vi "gyro-sweeper-server-V3.vi"(11 "talk to back IN":T4) -> ()   [LabVIEW 2018]
uses:
  cursor winow.ctl
  cursor window action.ctl
  KM_file -- read-write control.ctl
  filename-action.ctl
  file -- read-write control.ctl
  publisher action.ctl
  show-win- control.ctl
  data source action.ctl
  pll user action.ctl
  pll sweeper talkto message type.ctl
  pll sweeper talkback message type.ctl
  pll fitter talkto message type.ctl
  pll fitter talkback message type.ctl
  pll sweeper server talkto message type.ctl
  pll sweeper server talkback message type.ctl
  pll talkback message type.ctl
  filename-pattern.ctl
  talkto talkback pair.ctl
panel:
  out "Stop":bool
  in  "view/hide fitter async":bool
  in  "view/hide sweep async":bool
  in  "sweeper panel":T1(tab)
  in  "sweep ON":bool
  in  "win":T2={"cen (Hz)"=45005.0594236074, "win (Hz)"=127.23590686512762, "left (Hz)"=44941.44147017484, "right (Hz)"=45068.67737703997}
  out "Plot: circle sweep window":cluster{"Freq out (Hz)":dbl[], dbl[]}[](graph)
  in  "start/stop sweep: r":bool
  in  "subtract bgnd!":bool
  in  "fit!":bool=TRUE
  in  "cursor window":T3={"left"=2378.60310421286, "right "=2421.6740576496672, "center"=2421.6740576496672, "window"=2421.6740576496672, "cursors"=[], "relative"=0, "absolute"=0, "fixed vertical offset"=2421.6740576496672, "vertical offset"=2421.6740576496672, "skew"=2421.6740576496672, "default window frac"=2421.6740576496672, "kind"=enum."skewed", "skew.left"=2421.6740576496672, "skew.right"=2421.6740576496672, "Plot ref"=refnum, "wing order"=enum."back"}
  out "async sweeper reference out":refnum<vi>
  out "async fitter":refnum<vi>
  in  "save data":enum32{"save/read"}(tab)
  in  "freqsweep name template":T5={"prefix"="RuCl3-rod", "group"="f"}
  in  "Save folder":path=path "/Users/Shared/Data"
  in  "freq sweep file name":string="f020_RuCl3-rod_042518.dat"
  in  "read from disk :l":bool
  in  "read file":path=path "/Users/arkady/Desktop/local_data/TaAs-quirk-Jan2018-losalamos/9w/f006_rucl3_012518.dat"
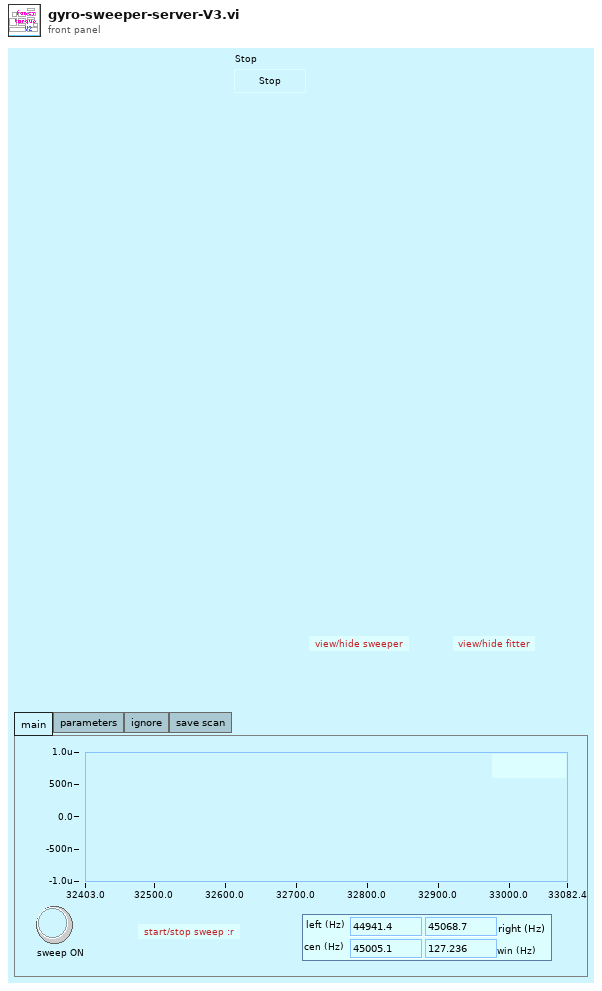
[diagram p1: front panel]
types:
  T1 = enum32{"main", "parameters", "ignore", "save scan"}
  T2 = typedef "show-win- control.ctl" = cluster{"cen (Hz)":dbl, "win (Hz)":dbl, "left (Hz)":dbl, "right (Hz)":dbl}
  T3 = typedef "cursor winow.ctl" = cluster{"left":dbl, "right ":dbl, "center":dbl, "window":dbl, "cursors":i32[], "relative":i32, "absolute":i32, "fixed vertical offset":dbl, "vertical offset":dbl, "skew":dbl, "default window frac":dbl, "kind":enum16{"symmetric", "skewed", "fancy"}, "skew.left":dbl, "skew.right":dbl, "Plot ref":refnum<vi>, "wing order":enum16{"forw", "back"}}
  T4 = typedef "talkto talkback pair.ctl" = cluster{"talkto event":refnum<user-event>, "talkback event":refnum<user-event>}
  T5 = typedef "filename-pattern.ctl" = cluster{"prefix":string, "group":string}
  T6 = cluster{"talkto event":refnum<user-event>, "talkback event":refnum<user-event>}
  T7 = typedef "pll fitter talkback message type.ctl" = cluster{"message":enum16{"new "}}
  T8 = typedef "pll fitter talkto message type.ctl" = cluster{"message":enum16{"stop", "start", "get new"}}
  T9 = typedef "data source action.ctl" = enum16{"set", "get", "init", "set-and-get", "init source"}
  T10 = typedef "pll sweeper talkback message type.ctl" = cluster{"message":enum16{"new"}}
  T11 = typedef "pll sweeper talkto message type.ctl" = cluster{"message":enum16{"stop", "start", "update pars"}}
  T12 = typedef "pll user action.ctl" = enum16{"fit"}
  T13 = typedef "publisher action.ctl" = enum16{"set", "get", "init", "check"}
  T14 = typedef "cursor window action.ctl" = enum16{"balance", "h. offset change", "cursor moves", "change center", "change window", "init", "check", "reset", "set y to middle", "idle", "-write all Y", "-write left.X", "-write center.X", "-write right.X", "-write all X", "-change center", "-change window", "-change skew", "-read cursor 2", "-read cursor 1", "-read cursor 0", "-read all cursors", "-reset", "-read plot scale", "-set y to middle", "-Q: center.Y is visible", "-Q: window is visible", "-parse center.Y", "-right left from center", "-left move", "-right move", "-set center.Y", "-empty", "-set cursors to default", "-check", "-write center.Y", "-copy cursor 1", "-copy cursor 0", "-copy cursor 2", "move right", "move left", "shrink", "broaden", "skew up", "skew down", "-write plot scale", "zoom X", "change cen&win", "zoom to all data", "color--red", "color--green", "color--yellow", "read", "zoom out", "zoom in", "slide right", "slide left", "set range aspect ratio to 1"}
  T15 = typedef "PLL data source.ctl" = enum16{"meta", "MFLI", "SRS865A"}
  T16 = typedef "file -- read-write control.ctl" = enum16{"read", "write all", "append one line"}
  T17 = typedef "filename-action.ctl" = enum16{"rewrite", "parse", "force pattern", "uniquenum"}
  T18 = typedef "KM_file -- read-write control.ctl" = enum16{"read", "write all", "append one line"}
  T19 = enum32{"Invalid", "Standard", "Closed", "Hidden", "Minimized", "Maximized"}
  T20 = typedef "eventvkey.ctl" = enum16{"ASCII", "Enter", "Return", "Shift", "Ctrl", "Alt", "Cmd", "Opt", "Caps", "NumLock", "Clear", "Break", "Up", "Down", "Left", "Right", "Insert", "Delete", "Home", "End", "PageUp", "PageDown", "Escape", "Help", "Pause", "ScrollLock", "F1", "F2", "F3", "F4", "F5", "F6", "F7", "F8", "F9", "F10", "F11", "F12", "F13", "F14", "F15", "F16", "F17", "F18", "F19", "F20", "F21", "F22", "F23", "F24", "Play", "VolumeUp", "VolumeDown", "Mute", "Two Byte Char"}
  T21 = typedef "pll talkback message type.ctl" = cluster{"message":enum16{"new", ""}}
  T22 = enum16{"exit", "parameter change", "start", "stop", "reset frequency", "reset lorentzian"}
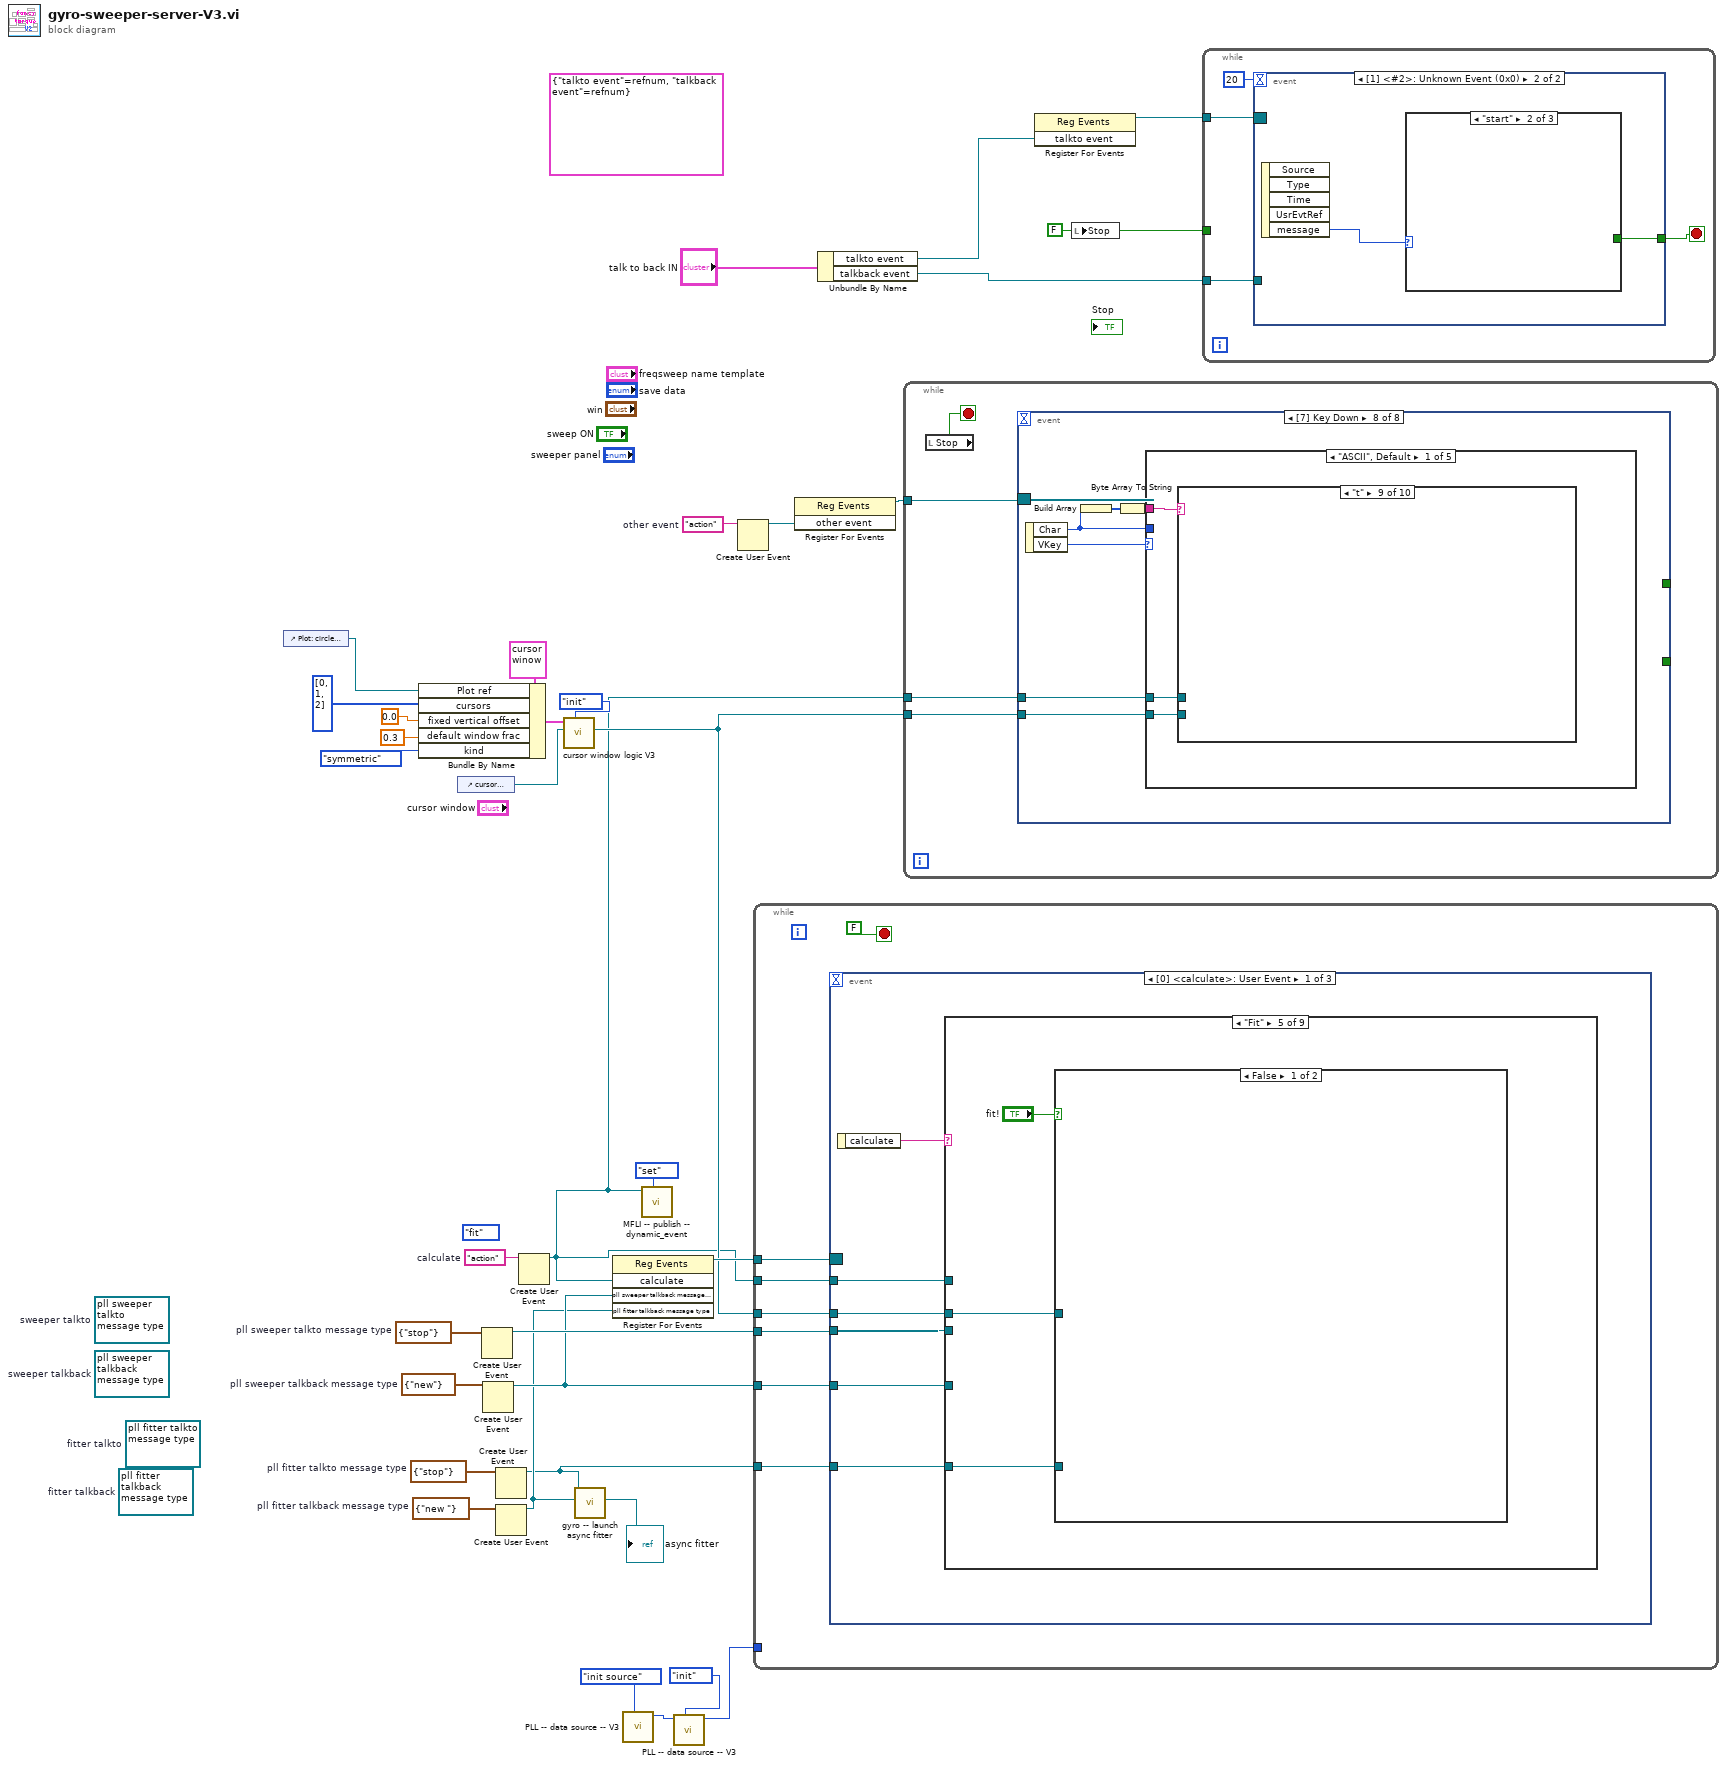
[diagram p0: block diagram]
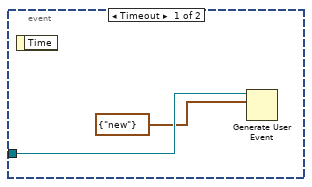
[diagram p2: hidden frame]
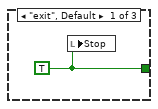
[diagram p3: hidden frame]
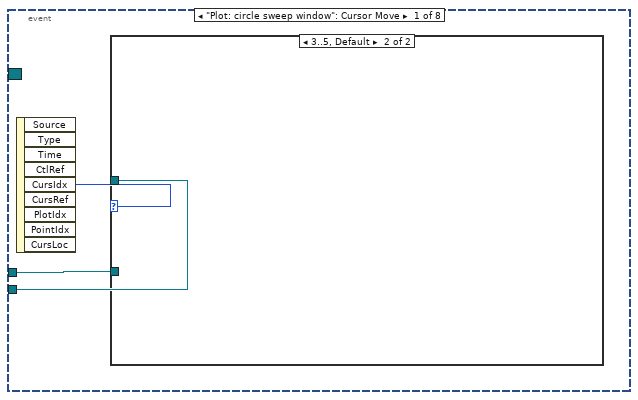
[diagram p5: hidden frame]
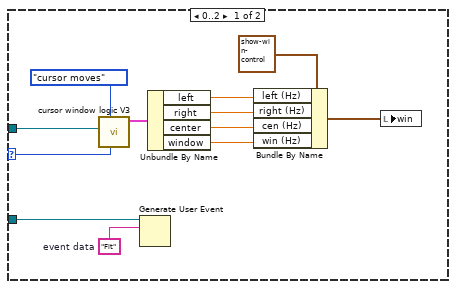
[diagram p6: hidden frame]
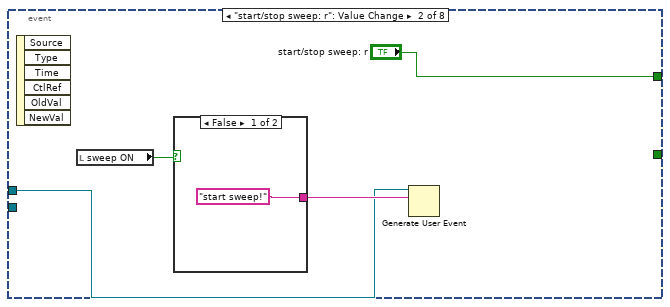
[diagram p7: hidden frame]
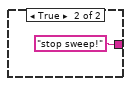
[diagram p8: hidden frame]
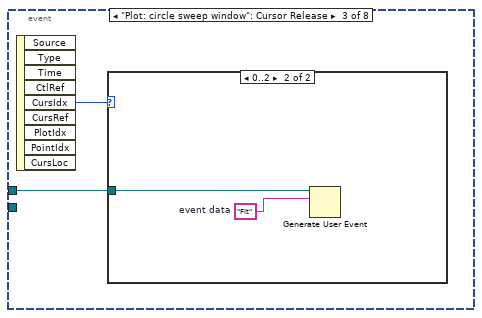
[diagram p9: hidden frame]
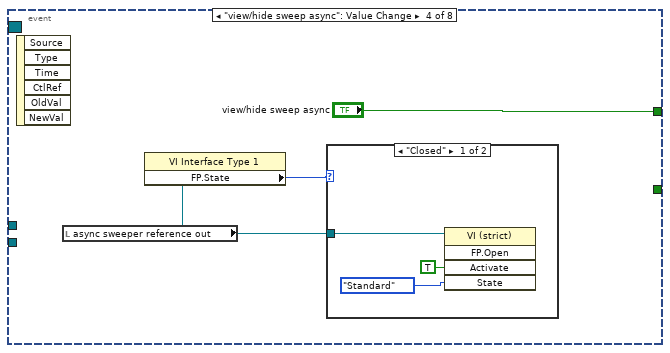
[diagram p11: hidden frame]
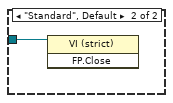
[diagram p12: hidden frame]
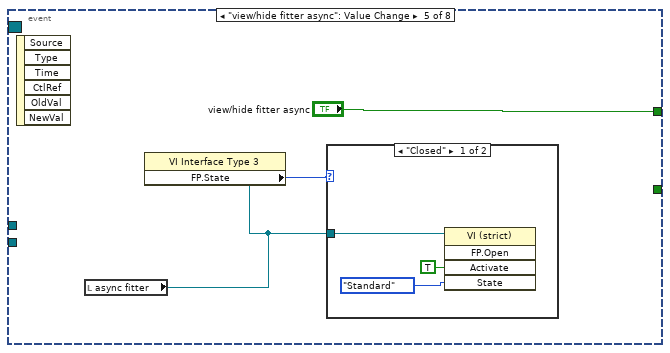
[diagram p13: hidden frame]
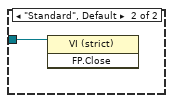
[diagram p14: hidden frame]
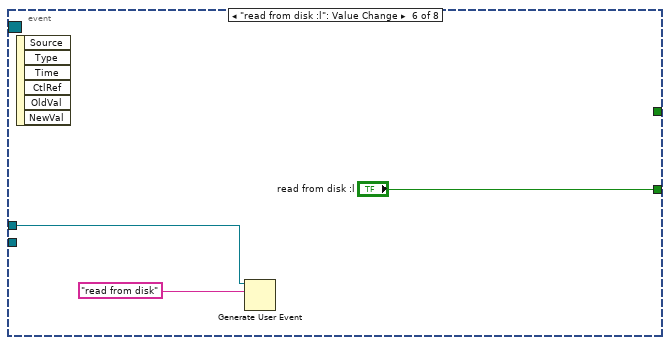
[diagram p15: hidden frame]
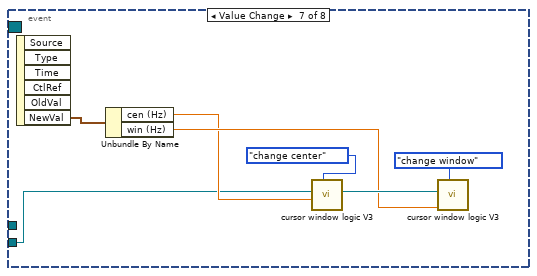
[diagram p16: hidden frame]
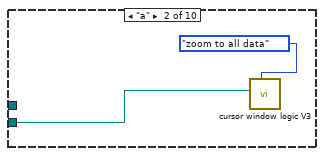
[diagram p18: hidden frame]
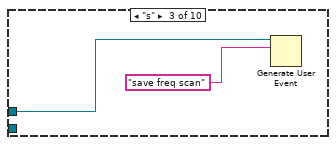
[diagram p19: hidden frame]
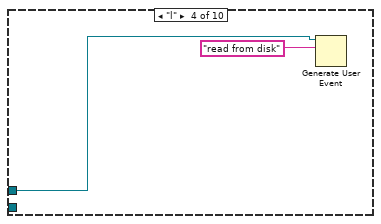
[diagram p20: hidden frame]
diagram:
  w4 = FALSE ("Stop")
  (unwired) T6 {"talkto event"=refnum, "talkback event"=refnum}
  (unwired) refnum<user-event> refnum  # fitter talkback
  (unwired) refnum<user-event> refnum  # fitter talkto
  w11 = T7 {"message"=enum."new "}  # pll fitter talkback message type
  w10 = T8 {"message"=enum."stop"}  # pll fitter talkto message type
  (unwired) refnum<user-event> refnum  # sweeper talkback
  (unwired) refnum<user-event> refnum  # sweeper talkto
  w19 = T10 {"message"=enum."new"}  # pll sweeper talkback message type
  w20 = T11 {"message"=enum."stop"}  # pll sweeper talkto message type
  (unwired) pll_user_action."fit" ("pll event action")
  w32 = "action"  # other event
  w34 = "action"  # calculate
  n1 = control-ref of="Plot: circle sweep window"() -> (w12:refnum<vi>)
  n2 = Bundle By Name(cluster=T3 {"left"=0.0, "right "=0.0, "center"=0.0, "window"=0.0, "cursors"=[], "relative"=0, "absolute"=0, "fixed vertical offset"=0.0, "vertical offset"=0.0, "skew"=0.0, "default window frac"=0.0, "kind"=enum."symmetric", "skew.left"=0.0, "skew.right"=0.0, "Plot ref"=refnum, "wing order"=enum."forw"} ("cursor bracket: All, data window"), "Plot ref"=w12, "cursors"=i32[] [0, 1, 2], "fixed vertical offset"=0.0, "default window frac"=0.3 ("fixed vertical offset"), "kind"=enum16{"symmetric", "skewed", "fancy"}."symmetric") -> (w26:T3)
  n3 = control-ref of="cursor window"() -> (w6:refnum<vi>)
  n4 = Create User Event(user event datatype=w20) -> (user event=w18:refnum<user-event>)  [unwired: 1 in, 1 out]
  n5 = Create User Event(user event datatype=w19) -> (user event=w16:refnum<user-event>)  [unwired: 1 in, 1 out]
  n6 = Create User Event(user event datatype=w10) -> (user event=w7:refnum<user-event>)  [unwired: 1 in, 1 out]
  n7 = Create User Event(user event datatype=w11) -> (user event=w8:refnum<user-event>)  [unwired: 1 in, 1 out]
  n8 = Create User Event(user event datatype=w34) -> (user event=w17:refnum<user-event>)  [unwired: 1 in, 1 out]
  n9 = call "cursor window logic V3.vi"("cursor window action"=cursor_window_action."init", "cursor window in"=w6, "cursor window init"=w26) -> ("cursor window out"=w22:refnum<vi>)  [unwired: 7 in, 1 out]
  n10 = call "gyro -- launch async fitter.vi"("fitter talkback"=w8, "fitter talkto"=w7) -> ("reference out"=→"async fitter":refnum<vi>)  [unwired: 9 in]
  n11 = register-events(w17, w16, w8) -> (reference out=w35:refnum<event-registration>)  [unwired: 2 in, 1 out]
  n12 = call "PLL -- data source -- V3.vi"("data source action"=data_source_action."init source") -> ("PLL data source OUT"=w15:T15)  [unwired: 8 in, 2 out]
  n13 = call "MFLI -- publish -- dynamic_event.vi"("publisher action"=publisher_action."set", "dynamic event"=w17) -> ()  [unwired: 9 in, 1 out]
  n14 = call "PLL -- data source -- V3.vi"("data source action"=data_source_action."init", "PLL data source"=w15) -> ("PLL data source OUT"=w14:T15)  [unwired: 7 in, 2 out]
  n15 = Create User Event(user event datatype=w32) -> (user event=w31:refnum<user-event>)  [unwired: 1 in, 1 out]
  n16 = while {
    tunnel: w35 -> [w42]
    tunnel: w17 -> [w40]
    tunnel: w22 -> [w39]
    tunnel: w14 -> [_]
    tunnel: w18 -> [w38]
    tunnel: w16 -> [w37]
    tunnel: w7 -> [w36]
    stop <- FALSE stop-if-true
    n17 = event shown="[0] <calculate>: User Event" {
      selector: w42 -> [_ _ _]
      dyn-events: _ -> [_ _ _]
      timeout: _ -> [_ _ _]
      tunnel: w40 -> [w47 w135 _]
      tunnel: w39 -> [w46 _ _]
      tunnel: w38 -> [w45 _ _]
      tunnel: w37 -> [w44 _ _]
      tunnel: w36 -> [w43 _ _]
      event User Event {
        n18 = event-data() -> ("calculate"=w48:string)  [unwired: 1 in]
        n19 = case shown="\"Fit\"" w48 {
          tunnel: w47 -> [w57 w79 w82 _ _ _ _ _ _]
          tunnel: w46 -> [_ _ _ _ w114 _ _ _ _]
          tunnel: w45 -> [_ _ _ _ _ w127 w130 w134 _]
          tunnel: w44 -> [_ _ _ _ _ w126 _ _ _]
          tunnel: w43 -> [_ _ _ _ w112 _ _ _ _]
          frame "New sweep data arrives" {
            n20 = call "MFLI -- publish -- freq scan.vi"("publisher action"=publisher_action."get") -> ("Voltage out (V)"=w54:cdb[], "Freq out (Hz)"=w56:dbl[])  [unwired: 9 in]
            n21 = Generate User Event(user event=w57, event data cluster="Fit" ("event data")) -> ()  [unwired: 2 in, 2 out]
            n22 = case shown="True" "subtract bgnd!" {
              tunnel: w56 -> [w69 w77]
              tunnel: [w63 w77] -> w55
              tunnel: w54 -> [w65 w76]
              tunnel: [w70 w76] -> w53
              frame True {
                w62 = 10 ("length")
                n23 = Delete From Array(array=w69, length=w62, index=0) -> (array with subset deleted=w68:dbl[])  [unwired: 1 out]
                n24 = Delete From Array(array=w65, length=w62, index=0) -> (array with subset deleted=w64:cdb[])  [unwired: 1 out]
                n25 = call "linear interp iiii- complex - z-omega.vi"("z"=w64, "omega"=w68) -> ("z out"=w71:cdb[], "omega out"=w63:dbl[], "intercept"=w73:cdb, "slope"=w74:cdb)  [unwired: 5 in, 5 out]
                n26 = Multiply(x=w63, y=w74) -> (x*y=w75:cdb[])
                n27 = Add(x=w75, y=w73) -> (x+y=w72:cdb[])
                n28 = Subtract(x=w71, y=w72) -> (x-y=w70:cdb[])
              }
              frame False {
              }
            }
            n29 = Complex To Re/Im(x + iy=w53) -> (x=w60:dbl[], y=w59:dbl[])
            n30 = Bundle("Freq out (Hz)"=w55, w60) -> (w61:cluster{"Freq out (Hz)":dbl[], dbl[]})  [unwired: 1 in]
            n31 = Bundle("Freq out (Hz)"=w55, w59) -> (w58:cluster{"Freq out (Hz)":dbl[], dbl[]})  [unwired: 1 in]
            n32 = Build Array(w61, w58) -> (→"Plot: circle sweep window":cluster{"Freq out (Hz)":dbl[], dbl[]}[])
          }
          frame "sweep off!" {
            n33 = local read "sweep ON"() -> (w78:bool)
            n34 = case shown="True" w78 {
              tunnel: w79 -> [_ w80]
              frame False {
              }
              frame True {
                n35 = Generate User Event(user event=w80, event data cluster="sweep!" ("event data")) -> ()  [unwired: 2 in, 2 out]
              }
            }
          }
          frame "read from disk" {
            n36 = call "file - read-write - list of lines.vi"("read/write control"=file_--_read-write_control."read", "file path"="read file") -> ("list of lines OUT"=w86:string[])  [unwired: 8 in, 1 out]
            n37 = for {
              tunnel: w86 -> [w96] mode=indexing
              tunnel: [w91] -> w87 mode=indexing
              tunnel: [w90] -> w88 mode=indexing
              w92 = 0.0
              n38 = Scan From String(format string="%f%f%f", input string=w96, default 1=w92, default 2=w92, default 3=w92) -> (output 1=w90:dbl, output 2=w94:dbl, output 3=w93:dbl)  [unwired: 2 in, 3 out]
              n39 = Re/Im To Complex(1:w93, 2:w94) -> (0:w91:cdb)
            }
            n40 = flat-sequence {
              tunnel: w82 -> [w100]
              tunnel: [w100] -> w89
              tunnel: w87 -> [w98]
              tunnel: w88 -> [w97]
              tunnel: w89 -> [w102]
              tunnel: "New sweep data arrives" ("event data") -> [w101]
              frame #0 {
                n41 = call "MFLI -- publish -- freq scan.vi"("publisher action"=publisher_action."set", "Voltage IN (V)"=w98, "Freq IN (Hz)"=w97) -> ()  [unwired: 7 in, 2 out]
              }
              frame #1 {
                n42 = Generate User Event(user event=w102, event data cluster=w101) -> ()  [unwired: 2 in, 2 out]
              }
            }
          }
          frame "save freq scan" {
            n43 = local read "freqsweep name template"() -> (w108:T5)
            n44 = call "MFLI -- publish -- freq scan.vi"("publisher action"=publisher_action."get") -> ("Voltage out (V)"=w104:cdb[], "Freq out (Hz)"=w105:dbl[])  [unwired: 9 in]
            n45 = call "filename-manage.vi"("filename pattern"=w108, "filename-action"=filename-action."uniquenum", "folder"="Save folder", "file name"="freq sweep file name") -> ("filename OUT"=w107:string)  [unwired: 7 in]
            n46 = call "KM_appendline -- freq sweep.vi"("freq"=w105, "Vout(V)"=w104, "Save frequency scan"="Save folder", "read/write control"=KM_file_--_read-write_control."append one line", "name or relative path"=w107) -> ()  [unwired: 15 in]
            n47 = local write "freq sweep file name"(w107) -> ()
          }
          frame "Fit" {
            n48 = case shown="False" "fit!" {
              tunnel: w114 -> [_ w116]
              tunnel: w112 -> [_ w115]
              frame False {
              }
              frame True {
                n49 = flat-sequence {
                  tunnel: w116 -> [w119]
                  tunnel: w115 -> [w122]
                  frame #0 {
                    n50 = call "cursor window logic V3.vi"("cursor window action"=cursor_window_action."read", "cursor window in"=w119) -> ("cursor window out"=w118:T3)  [unwired: 8 in, 1 out]
                    n51 = call "publish -- fitter window.vi"("publisher action"=publisher_action."set", "win IN"=w118) -> ()  [unwired: 9 in, 1 out]
                  }
                  frame #1 {
                    n52 = Generate User Event(user event=w122, event data cluster=T8 {"message"=enum."get new"} ("event data")) -> ()  [unwired: 2 in, 2 out]
                  }
                }
              }
            }
          }
          frame "start sweep!" {
            n53 = local read "win"() -> (w125:T2)
            n54 = local write "sweep ON"(TRUE ("sweep ON")) -> ()
            n55 = call "gyro -- launch async sweeper.vi"("win"=w125, "sweeper talkback"=w126, "sweeper talkto"=w127) -> ("reference out"=→"async sweeper reference out":refnum<vi>)  [unwired: 8 in]
          }
          frame "stop sweep!" {
            n56 = Generate User Event(user event=w130, event data cluster=T11 {"message"=enum."stop"} ("event data")) -> ()  [unwired: 2 in, 2 out]
            n57 = local write "sweep ON"(FALSE ("sweep ON")) -> ()
          }
          frame "update win" {
            n58 = local read "win"() -> (w131:T2)
            n59 = call "publish -- sweeper window.vi"("publisher action"=publisher_action."set", "win IN"=w131) -> ()  [unwired: 9 in, 1 out]
            n60 = Generate User Event(user event=w134, event data cluster=T11 {"message"=enum."update pars"} ("event data")) -> ()  [unwired: 2 in, 2 out]
          }
          frame "Void", Default {
          }
        }
      }
      event User Event {
        n61 = event-data() -> ("message"=w136:enum16{"new"})  [unwired: 1 in, 4 out]
        n62 = case shown="\"new\", Default" w136 {
          tunnel: w135 -> [w137]
          frame "new", Default {
            n63 = Generate User Event(user event=w137, event data cluster="New sweep data arrives" ("event data")) -> ()  [unwired: 2 in, 2 out]
          }
        }
      }
      event User Event {
        n64 = event-data() -> ()  [unwired: 1 in, 5 out]
      }
    }
  }
  n65 = register-events(w31) -> (reference out=w33:refnum<event-registration>)  [unwired: 2 in, 1 out]
  n66 = Unbundle By Name("talk to back IN") -> ("talkto event"=w3:refnum<user-event>, "talkback event"=w2:refnum<user-event>)
  n67 = while {
    tunnel: w33 -> [w142]
    tunnel: w17 -> [w141]
    tunnel: w22 -> [w140]
    stop <- w139 stop-if-true
    n68 = local read "Stop"() -> (w139:bool)
    n69 = event shown="[7] Key Down" {
      selector: w142 -> [_ _ _ _ _ _ _ _]
      dyn-events: _ -> [_ _ _ _ _ _ _ _]
      timeout: _ -> [_ _ _ _ _ _ _ _]
      tunnel: w141 -> [w143 w159 w165 _ _ w184 _ w196]
      tunnel: w140 -> [w145 _ _ _ _ _ w185 w192]
      tunnel: [_ "start/stop sweep: r" _ "view/hide sweep async" "view/hide fitter async" _ _ _] -> _
      tunnel: [_ _ _ _ _ "read from disk :l" _ _] -> _
      event "Plot: circle sweep window": Cursor Move {
        n70 = event-data() -> ("CursIdx"=w144:i32)  [unwired: 1 in, 8 out]
        n71 = case shown="3..5, Default" w144 {
          selector: w144 -> [w155 _]
          tunnel: w145 -> [w157 _]
          tunnel: w143 -> [w153 _]
          frame 0..2 {
            w152 = "Fit"  # event data
            n72 = call "cursor window logic V3.vi"("CursIdx"=w155, "cursor window action"=cursor_window_action."cursor moves", "cursor window in"=w157) -> ("cursor window out"=w154:T3)  [unwired: 7 in, 1 out]
            n73 = Generate User Event(user event=w153, event data cluster=w152) -> ()  [unwired: 2 in, 2 out]
            n74 = Unbundle By Name(w154) -> ("left"=w149:dbl, "right"=w148:dbl, "center"=w147:dbl, "window"=w146:dbl)
            n75 = Bundle By Name(cluster=T2 {"cen (Hz)"=-0.35260838541595674, "win (Hz)"=17.234446484426172, "left (Hz)"=-8.969831627629043, "right (Hz)"=8.26461485679713} ("win"), "left (Hz)"=w149, "right (Hz)"=w148, "cen (Hz)"=w147, "win (Hz)"=w146) -> (w150:T2)
            n76 = local write "win"(w150) -> ()
          }
          frame 3..5, Default {
          }
        }
      }
      event "start/stop sweep: r": Value Change {
        n77 = event-data() -> ()  [unwired: 1 in, 6 out]
        n78 = local read "sweep ON"() -> (w158:bool)
        n79 = case shown="False" w158 {
          tunnel: ["start sweep!" ("event data") "stop sweep!" ("event data")] -> w161
          frame False {
          }
          frame True {
          }
        }
        n80 = Generate User Event(user event=w159, event data cluster=w161) -> ()  [unwired: 2 in, 2 out]
      }
      event "Plot: circle sweep window": Cursor Release {
        n81 = event-data() -> ("CursIdx"=w164:i32)  [unwired: 1 in, 8 out]
        n82 = case shown="0..2" w164 {
          tunnel: w165 -> [_ w166]
          frame 3, Default {
          }
          frame 0..2 {
            w167 = "Fit"  # event data
            n83 = Generate User Event(user event=w166, event data cluster=w167) -> ()  [unwired: 2 in, 2 out]
          }
        }
      }
      event "view/hide sweep async": Value Change {
        n84 = event-data() -> ()  [unwired: 1 in, 6 out]
        n85 = local read "async sweeper reference out"() -> (w169:refnum<vi>)
        n86 = property class="VI Interface Type 1"(reference=w169) -> ("FP.State"=w170:T19)  [unwired: 1 in, 2 out]
        n87 = case shown="\"Closed\"" w170 {
          tunnel: w169 -> [w173 w174]
          frame "Closed" {
            n88 = invoke class="VI (strict)" method="FP.Open"(reference=w173, "Activate"=TRUE ("Activate?"), "State"=T19."Standard" ("Front Panel Window:State")) -> ()  [unwired: 2 in, 5 out]
          }
          frame "Standard", Default {
            n89 = invoke class="VI (strict)" method="FP.Close"(reference=w174) -> ()  [unwired: 2 in, 3 out]
          }
        }
      }
      event "view/hide fitter async": Value Change {
        n90 = event-data() -> ()  [unwired: 1 in, 6 out]
        n91 = local read "async fitter"() -> (w176:refnum<vi>)
        n92 = property class="VI Interface Type 3"(reference=w176) -> ("FP.State"=w177:T19)  [unwired: 1 in, 2 out]
        n93 = case shown="\"Closed\"" w177 {
          tunnel: w176 -> [w180 w181]
          frame "Closed" {
            n94 = invoke class="VI (strict)" method="FP.Open"(reference=w180, "Activate"=TRUE ("Activate?"), "State"=T19."Standard" ("Front Panel Window:State")) -> ()  [unwired: 2 in, 5 out]
          }
          frame "Standard", Default {
            n95 = invoke class="VI (strict)" method="FP.Close"(reference=w181) -> ()  [unwired: 2 in, 3 out]
          }
        }
      }
      event "read from disk :l": Value Change {
        n96 = event-data() -> ()  [unwired: 1 in, 6 out]
        n97 = Generate User Event(user event=w184, event data cluster="read from disk" ("event data")) -> ()  [unwired: 2 in, 2 out]
      }
      event Value Change {
        n98 = event-data() -> ("NewVal"=w188:T2)  [unwired: 1 in, 5 out]
        n99 = Unbundle By Name(w188) -> ("cen (Hz)"=w186:dbl, "win (Hz)"=w187:dbl)
        n100 = call "cursor window logic V3.vi"("cursor window action"=cursor_window_action."change center", "center"=w186, "cursor window in"=w185) -> ("cursor window out"=w189:refnum<vi>)  [unwired: 7 in, 1 out]
        n101 = call "cursor window logic V3.vi"("cursor window action"=cursor_window_action."change window", "window"=w187, "cursor window in"=w189) -> ()  [unwired: 7 in, 2 out]
      }
      event Key Down {
        n102 = event-data() -> ("Char"=w194:i16, "VKey"=w197:T20)  [unwired: 1 in]
        n103 = Build Array(w194) -> (w195:i16[])
        n104 = Byte Array To String(unsigned byte array=w195) -> (string=w193:string)
        n105 = case shown="\"ASCII\", Default" w197 {
          selector: w197 -> [_ _ _ _ w238]
          tunnel: w194 -> [_ _ _ _ _]
          tunnel: w196 -> [w200 _ _ _ w237]
          tunnel: w193 -> [w199 _ _ _ _]
          tunnel: w192 -> [w198 _ _ _ w234]
          frame "ASCII", Default {
            n106 = case shown="\"t\"" w199 {
              selector: w199 -> [_ _ _ _ _ _ w212 _ _ _]
              tunnel: w200 -> [_ _ w203 w205 w207 _ _ _ _ w221]
              tunnel: w198 -> [_ w201 _ _ _ w209 w213 w218 _ _]
              frame "0", Default {
              }
              frame "a" {
                n107 = call "cursor window logic V3.vi"("cursor window action"=cursor_window_action."zoom to all data", "cursor window in"=w201) -> ()  [unwired: 8 in, 2 out]
              }
              frame "s" {
                n108 = Generate User Event(user event=w203, event data cluster="save freq scan" ("event data")) -> ()  [unwired: 2 in, 2 out]
              }
              frame "l" {
                n109 = Generate User Event(user event=w205, event data cluster="read from disk" ("event data")) -> ()  [unwired: 2 in, 2 out]
              }
              frame "p" {
                n110 = Generate User Event(user event=w207, event data cluster="New sweep data arrives" ("event data")) -> ()  [unwired: 2 in, 2 out]
              }
              frame "?" {
                # "?"
                n111 = call "cursor window logic V3.vi"("cursor window action"=cursor_window_action."zoom X", "cursor window in"=w209) -> ()  [unwired: 8 in, 2 out]
              }
              frame "+", "-", "<", ">" {
                n112 = case shown="\"+\", Default" w212 {
                  tunnel: [cursor_window_action."slide right" ("cursor window action") cursor_window_action."slide left" ("cursor window action") cursor_window_action."zoom in" ("cursor window action") cursor_window_action."zoom out" ("cursor window action")] -> w211
                  frame ">" {
                  }
                  frame "<" {
                  }
                  frame "+", Default {
                  }
                  frame "-" {
                  }
                }
                n113 = call "cursor window logic V3.vi"("cursor window action"=w211, "cursor window in"=w213) -> ()  [unwired: 8 in, 2 out]
              }
              frame "c" {
                n114 = call "cursor window logic V3.vi"("cursor window action"=cursor_window_action."check", "cursor window in"=w218) -> ()  [unwired: 8 in, 2 out]
              }
              frame "t" {
              }
              frame "r" {
                n115 = local read "sweep ON"() -> (w220:bool)
                n116 = case shown="False" w220 {
                  tunnel: ["start sweep!" ("event data") "stop sweep!" ("event data")] -> w222
                  frame False {
                  }
                  frame True {
                  }
                }
                n117 = Generate User Event(user event=w221, event data cluster=w222) -> ()  [unwired: 2 in, 2 out]
              }
            }
          }
          frame "Escape" {
          }
          frame "PageUp" {
          }
          frame "PageDown" {
          }
          frame "Up".."Right" {
            w225 = "update win"  # event data
            w227 = "Fit"  # event data
            n118 = case shown="\"Left\"" w238 {
              tunnel: [cursor_window_action."move right" ("cursor window action") cursor_window_action."move left" ("cursor window action") cursor_window_action."broaden" ("cursor window action") cursor_window_action."shrink" ("cursor window action")] -> w236
              frame "Right", Default {
              }
              frame "Left" {
              }
              frame "Up" {
              }
              frame "Down" {
              }
            }
            n119 = call "cursor window logic V3.vi"("cursor window action"=w236, "cursor window in"=w234) -> ("cursor window out"=w235:T3)  [unwired: 8 in, 1 out]
            n120 = Unbundle By Name(w235) -> ("left"=w231:dbl, "right"=w230:dbl, "center"=w229:dbl, "window"=w228:dbl)
            n121 = Generate User Event(user event=w237, event data cluster=w227) -> (user event out=w226:refnum<user-event>)  [unwired: 2 in, 1 out]
            n122 = Bundle By Name(cluster=T2 {"cen (Hz)"=-0.35260838541595674, "win (Hz)"=17.234446484426172, "left (Hz)"=-8.969831627629043, "right (Hz)"=8.26461485679713} ("win"), "left (Hz)"=w231, "right (Hz)"=w230, "cen (Hz)"=w229, "win (Hz)"=w228) -> (w233:T2)
            n123 = Generate User Event(user event=w226, event data cluster=w225) -> ()  [unwired: 2 in, 2 out]
            n124 = local write "win"(w233) -> ()
          }
        }
      }
    }
  }
  n125 = register-events(w3) -> (reference out=w5:refnum<event-registration>)  [unwired: 2 in, 1 out]
  n126 = local write "Stop"(w4) -> ()
  n127 = while {
    tunnel: w5 -> [w246]
    tunnel: w2 -> [w244]
    tunnel: w4 -> [_]
    stop <- w243 stop-if-true
    n128 = event shown="[1] <#2>: Unknown Event (0x0)" {
      selector: w246 -> [_ _]
      dyn-events: _ -> [_ _]
      timeout: 20 -> [_ _]
      tunnel: w244 -> [w248 _]
      tunnel: [_ w249] -> w243
      event Timeout {
        n129 = event-data() -> ()  [unwired: 1 in, 1 out]
        n130 = Generate User Event(user event=w248, event data cluster=T21 {"message"=enum."new"} ("event data")) -> ()  [unwired: 2 in, 2 out]
      }
      event User Event {
        n131 = event-data() -> ("message"=w250:T22)  [unwired: 1 in, 4 out]
        n132 = case shown="\"start\"" w250 {
          tunnel: [w251 _ _] -> w249
          frame "exit", Default {
            w251 = TRUE
            n133 = local write "Stop"(w251) -> ()
          }
          frame "start" {
          }
          frame "stop" {
          }
        }
      }
    }
  }
